vi "conj_block.vi"(2 "Control":T3, 3 "B":T4, 4 "A":T5) -> (0 "Flags":T1, 1 "Result":T2)   [LabVIEW 2013]
panel:
  # "R1"
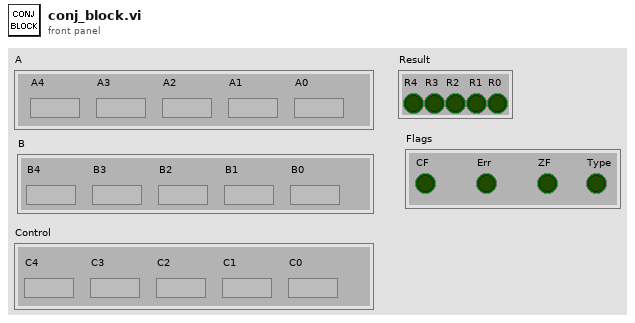
[diagram p1: front panel]
types:
  T1 = cluster{"CF":bool, "Err":bool, "ZF":bool, "Type":bool}
  T2 = cluster{"R4":bool, "R3":bool, "R2":bool, bool, "R0":bool}
  T3 = cluster{"C4":bool, "C3":bool, "C2":bool, "C1":bool, "C0":bool}
  T4 = cluster{"B4":bool, "B3":bool, "B2":bool, "B1":bool, "B0":bool}
  T5 = cluster{"A4":bool, "A3":bool, "A2":bool, "A1":bool, "A0":bool}
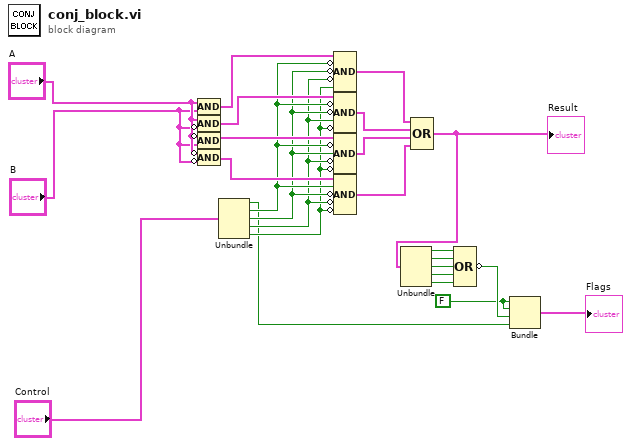
[diagram p0: block diagram]
diagram:
  w3 = FALSE
  n1 = Compound Arithmetic op=AND("A", "B") -> (w23:cluster{bool, bool, bool, bool, bool})
  n2 = Compound Arithmetic op=AND("A", invert "B") -> (w22:cluster{bool, bool, bool, bool, bool})
  n3 = Compound Arithmetic op=AND(invert "A", "B") -> (w21:cluster{bool, bool, bool, bool, bool})
  n4 = Compound Arithmetic op=AND(invert "A", invert "B") -> (w20:cluster{bool, bool, bool, bool, bool})
  n5 = Unbundle("Control") -> ("C4"=w1:bool, "C3"=w15:bool, "C2"=w14:bool, "C1"=w13:bool, "C0"=w12:bool)
  n6 = Compound Arithmetic op=AND(w23, invert w15, invert w14, invert w13, w12) -> (w19:cluster{bool, bool, bool, bool, bool})
  n7 = Compound Arithmetic op=AND(w22, invert w15, invert w14, w13, invert w12) -> (w18:cluster{bool, bool, bool, bool, bool})
  n8 = Compound Arithmetic op=AND(w21, invert w15, w14, invert w13, invert w12) -> (w17:cluster{bool, bool, bool, bool, bool})
  n9 = Compound Arithmetic op=AND(w20, w15, invert w14, invert w13, invert w12) -> (w16:cluster{bool, bool, bool, bool, bool})
  n10 = Compound Arithmetic op=OR(w19, w18, w17, w16) -> (w10:cluster{bool, bool, bool, bool, bool})
  "Result" <- w10
  n11 = Unbundle(w10) -> (w9:bool, w8:bool, w7:bool, w6:bool, w5:bool)
  n12 = Compound Arithmetic op=OR(w9, w8, w7, w6, w5) -> (invert w4:bool)
  n13 = Bundle(w3, w3, w4, "C4"=w1) -> (→"Flags":cluster{bool, bool, bool, "C4":bool})  [unwired: 1 in]
